vi "ActionVIDebug.vi"(11 "Compiled.Settings":T1) -> ()   [LabVIEW 2016, in "DDS Custom Device System Explorer.lvlib"]
uses:
  DDS Custom Device System Explorer.lvlib
  Shared/Compiled.Settings.ctl
  Shared/WriterReaderConfiguration.ctl
  Shared/Advanced DDS Configuration.ctl
  Shared/key Enum.ctl
  <vilib>/RTI DDS Toolkit/Types/RTI DDS ContentFilteredTopic Info.ctl
  <vilib>/RTI DDS Toolkit/Library/LVDDS_library.lvlib
  Shared/DDS Custom Device Shared.lvlib
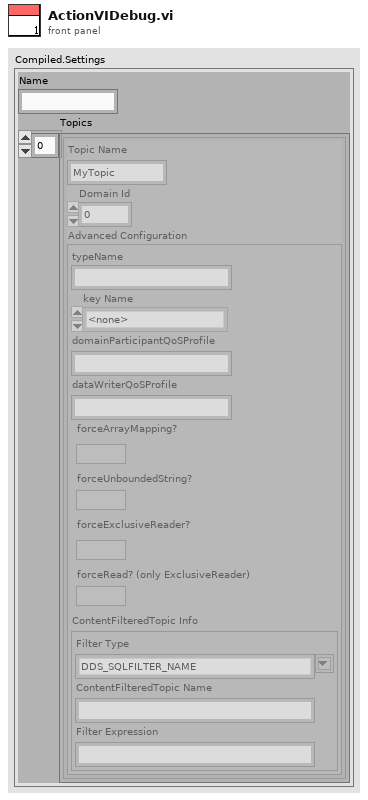
[diagram p1: front panel]
types:
  T1 = typedef "DDS Custom Device Shared.lvlib/Compiled.Settings.ctl" = cluster{"Name":string, "Topics":T2[]}
  T2 = typedef "DDS Custom Device Shared.lvlib/WriterReaderConfiguration.ctl" = cluster{"Topic Name":string, "Domain Id":u32, "Advanced Configuration":T3}
  T3 = typedef "DDS Custom Device Shared.lvlib/Advanced DDS Configuration.ctl" = cluster{"typeName":string, "key Name":T4, "domainParticipantQoSProfile":string, "dataWriterQoSProfile":string, "forceArrayMapping?":bool, "forceUnboundedString?":bool, "forceExclusiveReader?":bool, "forceRead? (only ExclusiveReader)":bool, "ContentFilteredTopic Info":T5}
  T4 = typedef "DDS Custom Device Shared.lvlib/key Enum.ctl" = enum16{"<none>", "I32_Num", "I64_Num", "U16_Num", "innercluster.Sgl_Num", "innercluster.Boolean"}
  T5 = typedef "LVDDS_library.lvlib/RTI DDS ContentFilteredTopic Info.ctl" = cluster{"Filter Type":string, "ContentFilteredTopic Name":string, "Filter Expression":string}
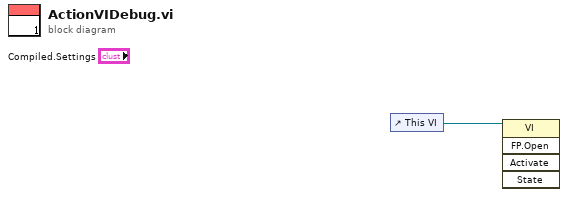
[diagram p0: block diagram]
diagram:
  n1 = control-ref of="This VI"() -> (w1:refnum<vi>)
  n2 = invoke class="VI" method="FP.Open"(reference=w1) -> ()  [unwired: 4 in, 5 out]
